vi "Trial Config - Load Filenames.vi"(8 "Error IN":errorcluster) -> (0 "Error OUT":errorcluster, 3 "Trial Config File Names OUT":string[](array[string]))   [LabVIEW 2018]
uses:
  Globals/Global - Configuration Options.vi
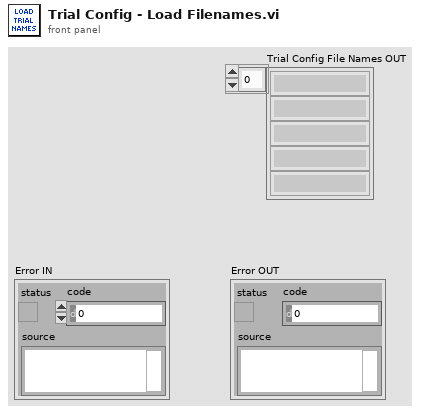
[diagram p1: front panel]
types:
  T1 = typedef "Rig Config Settings.ctl" = cluster{"Rig Name":string, "Rig Room":string, "Base Directory":string, "Computer IP Address":string, "Globals Name":string, "Treatmill Str":string, "cRIO Test Data Dir":path, "ai":string, "ao":string, "dio":string, "A_calib_str_row1":string, "A_calib_str_row2":string, "A_calib_str_row3":string, "Zero_V_str":string, "step_V":string, "Sample Freq":string, "ai_threshold":string, "run_speed_thresh":string, "speed_time_length":string, "wall ball gain":string, "max wall pos":string, "max cor width":string, "Trial Config Directory":path, "Randomize Trials?":bool}
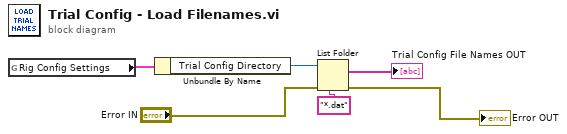
[diagram p0: block diagram]
diagram:
  n1 = global read "Global - Configuration Options.vi" "Rig Config Settings"() -> (w3:T1)
  n2 = Unbundle By Name(w3) -> ("Trial Config Directory"=w5:path)
  n3 = List Folder(path=w5, pattern="*.dat", error in="Error IN") -> (filenames=→"Trial Config File Names OUT":string[], error out=→"Error OUT":errorcluster)  [unwired: 1 in, 2 out]
